vi "Write Current States.vi"(8 "error in (no error)":errorcluster, 10 "Enum":T1=enum."IncreaseVoltage", 11 "ChirpEIS in":refnum<class "ChirpEIS.lvclass">) -> (0 "error out":errorcluster, 2 "Boolean":bool=TRUE, 3 "ChirpEIS out":refnum<class "ChirpEIS.lvclass">)   [LabVIEW 2014, in "ChirpEIS.lvclass"]
uses:
  ChirpEIS.lvclass
  States.ctl
  ChirpEIS.lvclass/ChirpEIS.ctl
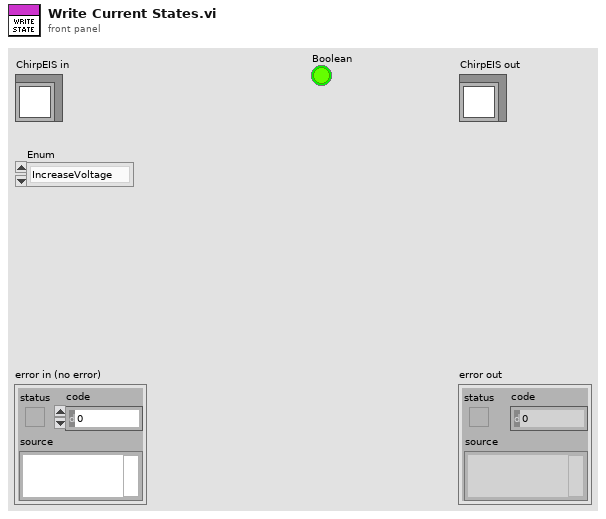
[diagram p1: front panel]
types:
  T1 = typedef "States.ctl" = enum16{"AddDuration", "AddFreq", "CreateNewFile", "Wait", "IncreaseVoltage", "DFT", "ChirpMeasurement", "Initialize", "Ternimate"}
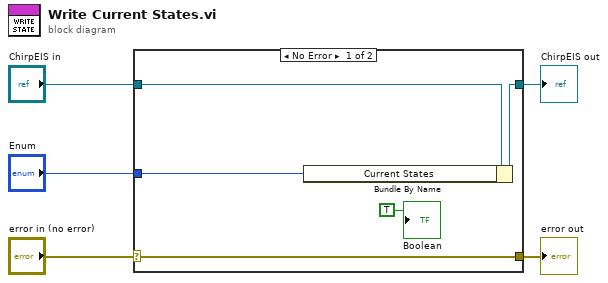
[diagram p0: block diagram]
diagram:
  n1 = case shown="No Error" "error in (no error)" {
    selector: "error in (no error)" -> [w10 w11]
    tunnel: [w10 w11] -> w4
    tunnel: [w8 w12] -> w2
    tunnel: "ChirpEIS in" -> [w9 w12]
    tunnel: "Enum" -> [w7 _]
    frame No Error {
      n2 = Bundle By Name(cluster=w9, "Current States"=w7) -> (w8:refnum<class "ChirpEIS.lvclass">)
      "Boolean" <- TRUE
    }
    frame Error {
    }
  }
  "error out" <- w4
  "ChirpEIS out" <- w2
